vi "testthisout.vi"() -> ()   [LabVIEW 2012]
panel:
  in  "Wave Number":u16(slide) scale=0.0..2.0
  in  "OK Button":bool
  in  "stop":bool
  out "output array":T1(array[cluster])
  in  "Cluster":T2={"Specimen 2"="", "Location 2"="", "Species 2"="", "Temp 2"="", "Comments 2"="", "Gain 2"=0.0, "Coupling 2"=TRUE, "Date 2"="", "Time 2"=""} {"Gain 2" items=["10"=10.0, "20"=20.0, "50"=50.0, "100"=100.0, "200"=200.0, "500"=500.0, "1k"=1000.0, "2k"=2000.0, "5k"=5000.0, "10k"=10000.0, "20k"=20000.0, "50k"=50000.0]}
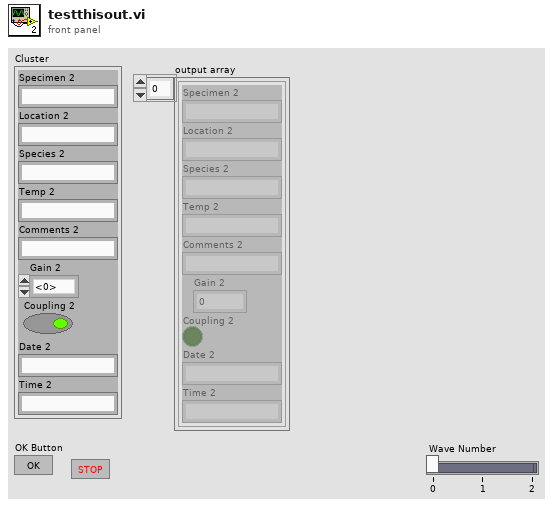
[diagram p1: front panel]
types:
  T1 = cluster{"Specimen 2":string, "Location 2":string, "Species 2":string, "Temp 2":string, "Comments 2":string, "Gain 2":dbl, "Coupling 2":bool, "Date 2":string, "Time 2":string}[]
  T2 = cluster{"Specimen 2":string, "Location 2":string, "Species 2":string, "Temp 2":string, "Comments 2":string, "Gain 2":dbl, "Coupling 2":bool, "Date 2":string, "Time 2":string}
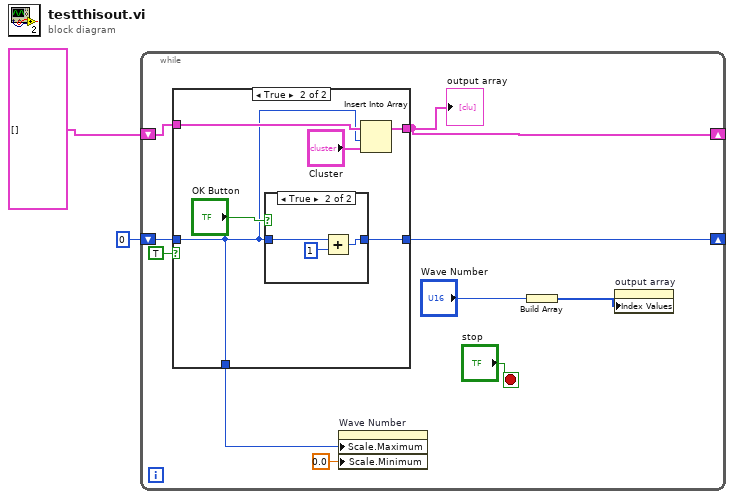
[diagram p0: block diagram]
diagram:
  n1 = while {
    shift-right: [w11] -> _
    shift-left: 0 -> [w10]
    shift-right: [w8] -> _
    shift-left: T1 [] ("output array 2") -> [w7]
    stop <- "stop" stop-if-true
    n2 = case shown="True" TRUE {
      tunnel: w10 -> [_ w13]
      tunnel: [_ w17] -> w11
      tunnel: [_ w16] -> w8
      tunnel: w7 -> [_ w14]
      tunnel: [_ w13] -> w4
      frame False {
      }
      frame True {
        n3 = case shown="True" "OK Button" {
          tunnel: [w19 w21] -> w17
          tunnel: w13 -> [w19 w20]
          frame False {
          }
          frame True {
            n4 = Add(x=w20, y=1) -> (x+y=w21:i32)
          }
        }
        n5 = Insert Into Array(array=w14, index=w13, new element="Cluster") -> (w16:T1)
      }
    }
    "output array" <- w8
    n6 = property on="Wave Number" class="Slide (strict)"("Scale.Maximum"=w4, "Scale.Minimum"=0.0 ("Scale.Range:Minimum")) -> ()  [unwired: 2 in, 2 out]
    n7 = Build Array("Wave Number") -> (w5:u16[])
    n8 = property on="output array" class="Arr (strict)"("Index Values"=w5) -> ()  [unwired: 2 in, 2 out]
  }
